vi "Get UUT Serial Port Parameters.vi"(0 "VISA resource name":refnum<visa-resource-name>, 11 "error in (no error)":errorcluster) -> (3 "Baud Rate":i32, 4 "VISA resource name out":refnum<visa-resource-name>, 6 "Flow Control":i32, 8 "Number Data Bits":i32, 10 "Number Stop Bits":i32, 14 "Parity":i32, 15 "error out":errorcluster)   [LabVIEW 2011, in "Fluke 5XXX Series Multicalibrators.lvlib"]
doc: "This VI returns the RS-232-C settings for the Calibrator rear panel SERIAL 2 TO UUT serial port.\n\nNote:\n\nThis VI is available only for instrument models 5500A and 5520A."
uses:
  Fluke 5XXX Series Multicalibrators.lvlib
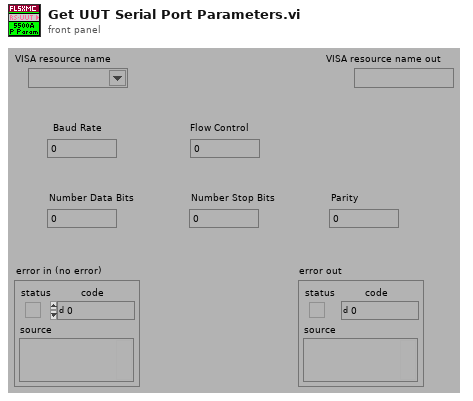
[diagram p1: front panel]
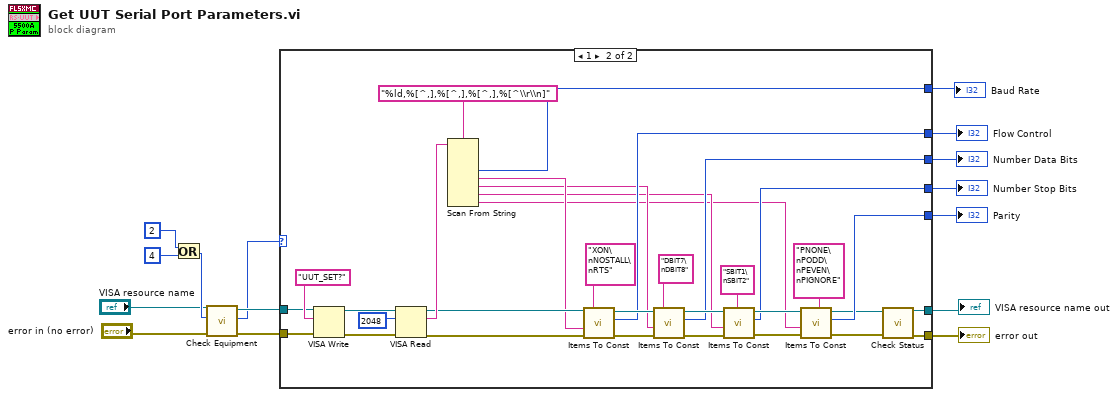
[diagram p0: block diagram]
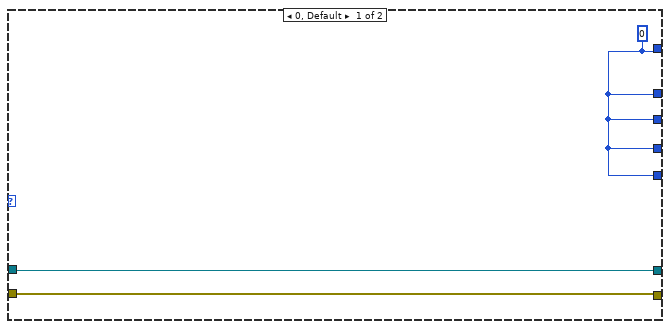
[diagram p2: hidden frame]
diagram:
  n1 = Or(x=2 ("Numeric"), y=4 ("Numeric")) -> (x .or. y?=w11:i32)
  n2 = call "Check Equipment.vi"("error in (no error)"="error in (no error)", "Bit Mask"=w11, "VISA resource name"="VISA resource name") -> ("error out"=w9:errorcluster, "Present?"=w6:u32, "VISA resource name out"=w7:refnum<visa-resource-name>)  [unwired: 6 in]
  n3 = case shown="1" w6 {
    tunnel: [w18 w35] -> w15
    tunnel: [w17 w34] -> w14
    tunnel: w9 -> [w18 w33]
    tunnel: w7 -> [w17 w32]
    tunnel: [w16 w31] -> w5
    tunnel: [w16 w30] -> w4
    tunnel: [w16 w29] -> w3
    tunnel: [w16 w28] -> w2
    tunnel: [w16 w27] -> w1
    frame 0, Default {
      w16 = 0
    }
    frame 1 {
      n4 = VISA Write(VISA resource name=w32, write buffer="UUT_SET?", error in (no error)=w33) -> (VISA resource name out=w50:refnum<visa-resource-name>, error out=w49:errorcluster)  [unwired: 1 out]
      n5 = VISA Read(VISA resource name=w50, byte count=u32 2048 ("byte count (0)"), error in (no error)=w49) -> (VISA resource name out=w24:refnum<visa-resource-name>, read buffer=w46:string, error out=w23:errorcluster)  [unwired: 1 out]
      n6 = Scan From String(format string="%ld,%[^,],%[^,],%[^,],%[^\\r\\n]", input string=w46) -> (output 1=w31:i32, output 2=w22:string, output 3=w21:string, output 4=w20:string, output 5=w19:string)  [unwired: 7 in, 3 out]
      n7 = call "Items To Const.vi"("error in (no error)"=w23, "String Item"=w22, "Multi-Line String"="XON\nNOSTALL\nRTS" ("Reset Command"), "VISA resource name"=w24) -> ("error out"=w45:errorcluster, "Index"=w30:i32, "VISA resource name out"=w42:refnum<visa-resource-name>)  [unwired: 5 in]
      n8 = call "Items To Const.vi"("error in (no error)"=w45, "String Item"=w21, "Multi-Line String"="DBIT7\nDBIT8" ("Reset Command"), "VISA resource name"=w42) -> ("error out"=w44:errorcluster, "Index"=w29:i32, "VISA resource name out"=w41:refnum<visa-resource-name>)  [unwired: 5 in]
      n9 = call "Items To Const.vi"("error in (no error)"=w44, "String Item"=w20, "Multi-Line String"="SBIT1\nSBIT2" ("Reset Command"), "VISA resource name"=w41) -> ("error out"=w43:errorcluster, "Index"=w28:i32, "VISA resource name out"=w40:refnum<visa-resource-name>)  [unwired: 5 in]
      n10 = call "Items To Const.vi"("error in (no error)"=w43, "String Item"=w19, "Multi-Line String"="PNONE\nPODD\nPEVEN\nPIGNORE" ("Reset Command"), "VISA resource name"=w40) -> ("error out"=w26:errorcluster, "Index"=w27:i32, "VISA resource name out"=w25:refnum<visa-resource-name>)  [unwired: 5 in]
      n11 = call "Check Status.vi"("VISA resource name"=w25, "error in (no error)"=w26) -> ("VISA resource name out"=w34:refnum<visa-resource-name>, "error out"=w35:errorcluster)  [unwired: 12 in]
    }
  }
  "Baud Rate" <- w5
  "Flow Control" <- w4
  "Number Data Bits" <- w3
  "Number Stop Bits" <- w2
  "Parity" <- w1
  "VISA resource name out" <- w14
  "error out" <- w15
